vi "Periodic Tasks.vi"(8 "error in":errorcluster) -> ()   [LabVIEW 2018]
doc: "This VI runs in parallel to other tasks. It can contain as many user-defined periodic loops as you need. These can carry out PID or other sorts of timed response."
uses:
  <vilib>/Rock Robotics/WPI/Utilities/WPI_GetSetVariantRefNum.vi
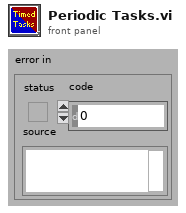
[diagram p1: front panel]
types:
  T1 = typedef "WPI_CompressorDevRef.ctl" = cluster{"DevStatus":errorcluster, "Pneumatics Control Module":u8}
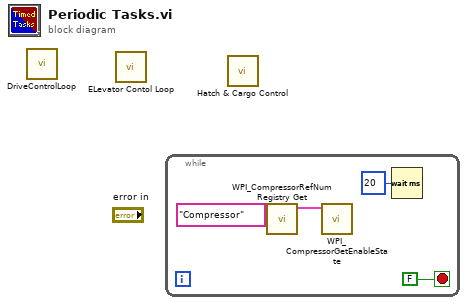
[diagram p0: block diagram]
diagram:
  n1 = call "DriveControlLoop.vi"() -> ()  [unwired: 12 in]
  n2 = call "ELevator Contol Loop.vi"() -> ()  [unwired: 12 in]
  n3 = while {
    stop <- FALSE stop-if-true
    n4 = call <vilib>:"WPI_CompressorRefNum Registry Get.vi"("refnum name"="Compressor") -> ("CompressorDevRef"=w1:T1)  [unwired: 9 in, 1 out]
    n5 = call <vilib>:"WPI_CompressorGetEnableState.vi"("CompressorDevRef"=w1) -> ()  [unwired: 7 in, 4 out]
    n6 = Wait (ms)(milliseconds to wait=u32 20) -> ()  [unwired: 1 out]
  }
  n7 = call "Hatch & Cargo Control.vi"() -> ()  [unwired: 12 in]
